vi "Send.vi"(8 "error in":errorcluster, 11 "Upload Transfer in":refnum<class "Upload Transfer.lvclass">) -> (0 "error out":errorcluster, 3 "Upload Transfer out":refnum<class "Upload Transfer.lvclass">)   [LabVIEW 2020, in "SDO Manager.lvlib" / "Upload Transfer.lvclass"]
doc: "Service SDO upload\nThe client is using the service SDO upload for transferring the data from the server (owner of the\nobject dictionary) to the client."
uses:
  Upload Transfer.lvclass
  HAL/Source/Interfaces/ICommunicate/ICommunicate.lvclass
  CANopen Message/CANopen Message.lvclass
  Upload Transfer.lvclass/Upload Transfer.ctl
  Typedefs/Function Code.ctl
  CANopen.lvlib
  SDO Transfer/SDO Transfer.lvclass
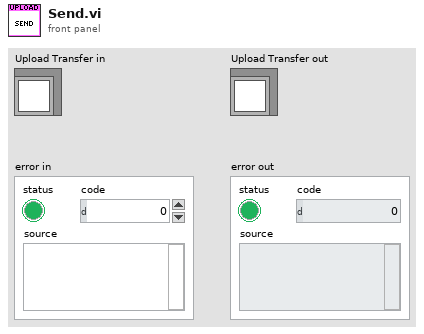
[diagram p1: front panel]
types:
  T1 = typedef "CANopen.lvlib/Function Code.ctl" = u8
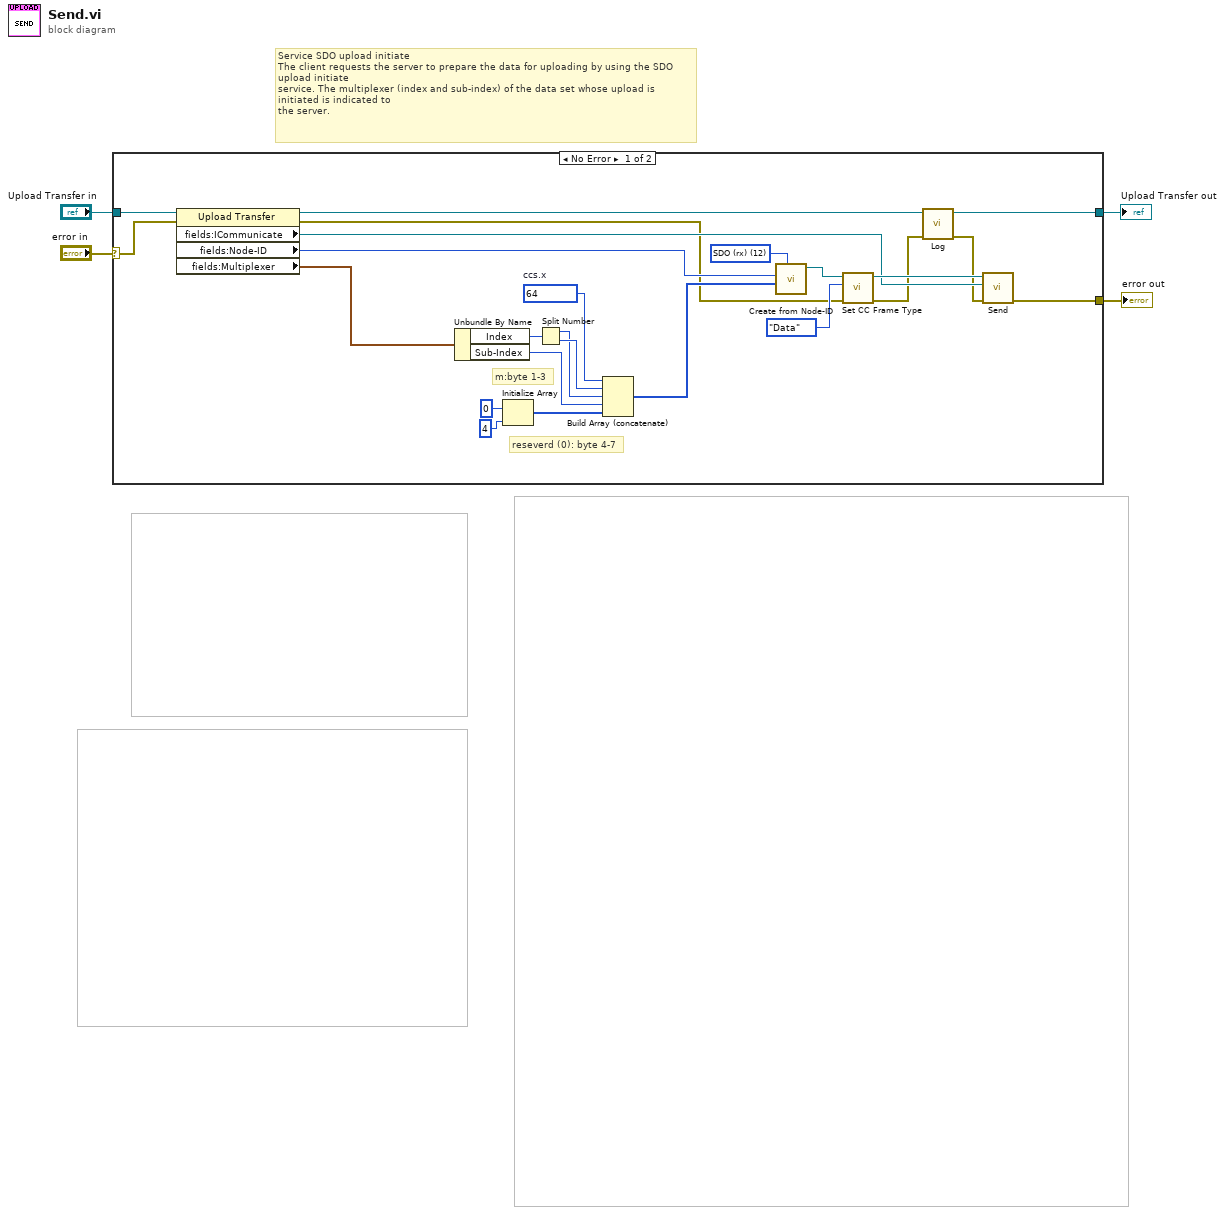
[diagram p0: block diagram]
diagram:
  # "Service SDO upload initiate\nThe client requests the server to prepare the data for uploading by using the SDO upload initiate\nservice. The multiplexer (index and sub-index) of the data set whose upload is initiated is indicated to\nthe server."
  n1 = case shown="No Error" "error in" {
    selector: "error in" -> [w28 w29]
    tunnel: "Upload Transfer in" -> [w27 w30]
    tunnel: [w9 w30] -> w2
    tunnel: [w8 w29] -> w1
    frame No Error {
      w16 = T1 12 items=["NMT"=0, "EMCY/SYNC"=1, "TIME"=2, "PDO1 (tx)"=3, "PDO1 (rx)"=4, "PDO2 (tx)"=5, "PDO2 (rx)"=6, "PDO3 (tx)"=7, "PDO3 (rx)"=8, "PDO4 (tx)"=9, "PDO4 (rx)"=10, "SDO (tx)"=11, "SDO (rx)"=12, "NMT error control"=14] ("Function Code")
      w21 = u8 64  # ccs.x
      # "reseverd (0): byte 4-7"
      # "m:byte 1-3"
      n2 = property class="Upload Transfer"(reference=w27, error in=w28) -> (reference out=w10:refnum<class "Upload Transfer.lvclass">, error out=w7:errorcluster, "fields:ICommunicate"=w11:refnum<class "ICommunicate.lvclass">, "fields:Node-ID"=w26:u8, "fields:Multiplexer"=w18:cluster{"Index":u16, "Sub-Index":u8})
      n3 = Unbundle By Name(w18) -> ("Index"=w25:u16, "Sub-Index"=w22:u8)
      n4 = Initialize Array(u8 0, 4 ("y")) -> (w20:u8[])
      n5 = Split Number(x=w25) -> (hi(x)=w23:u8, lo(x)=w24:u8)
      n6 = Build Array (concatenate)(w21, w24, w23, w22, w20) -> (w17:u8[])
      n7 = call "Create from Node-ID.vi"("Function Code"=w16, "Data"=w17, "Node-ID"=w26) -> ("CANopen Message"=w15:refnum<class "CANopen Message.lvclass">)  [unwired: 8 in]
      n8 = call "Set CC Frame Type.vi"("error in"=w7, "CC Frame Type"=enum8{"Data", "Remote", "Error", "Overload"}."Data", "CANopen Message in"=w15) -> ("error out"=w6:errorcluster, "CANopen Message out"=w14:refnum<class "CANopen Message.lvclass">)  [unwired: 7 in]
      n9 = call "Log.vi"("error in"=w6, "SDO Transfer in"=w10) -> ("error out"=w5:errorcluster, "SDO Transfer out"=w9:refnum<class "Upload Transfer.lvclass">)  [unwired: 8 in]
      n10 = call "Send.vi"("error in"=w5, "ICommunicate"=w11, "CANopen Message in"=w14) -> ("error out"=w8:errorcluster)  [unwired: 7 in, 1 out]
    }
    frame Error {
    }
  }
  "Upload Transfer out" <- w2
  "error out" <- w1
